vi "AD5933_ReadFrequencySweepValues (NI-845x I2C)(SubVI).vi"(7 "error in":errorcluster, 9 "ConfigRegister (0x80)":u8, 10 "NI-845x Config for I2C (in)":cluster{"i2c configuration":T1, "Refnum in":T2}) -> (0 "error out":errorcluster, 1 "I Array":i16[](array[numeric]), 2 "R Array":i16[](array[numeric]), 3 "NI-845x Config for I2C (out)":T3)   [LabVIEW 2017]
uses:
  <vilib>/ni845x/ni845x.llb/ni845xI2cConfiguration.ctl
  <vilib>/ni845x/ni845x.llb/ni845xControl.ctl
  TypeDefs/AD5933_CommandCodes.ctl
  TypeDefs/AD5933_Registers.ctl
  TypeDefs/AD5933_OperationState.ctl
  <vilib>/MakerHub/Toolbox/LMH-Toolbox.lvlib
panel:
  out "Frequency sweep complete":bool
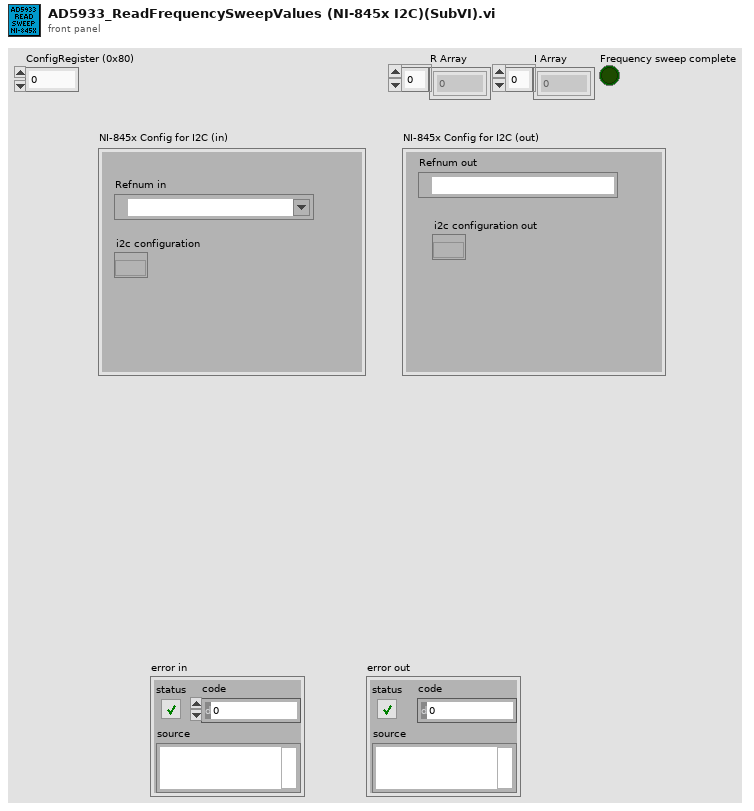
[diagram p1: front panel]
types:
  T1 = typedef "ni845xI2cConfiguration.ctl" = refnum<k20>
  T2 = typedef "ni845xControl.ctl" = refnum<k21>
  T3 = cluster{"i2c configuration out":T1, "Refnum out":T2}
  T4 = cluster{"Valid temperature measurement":bool, "Valid real/imaginary data":bool, "Frequency sweep complete":bool}
  T5 = typedef "AD5933_CommandCodes.ctl" = u8
  T6 = typedef "AD5933_Registers.ctl" = u8
  T7 = typedef "AD5933_OperationState.ctl" = u8
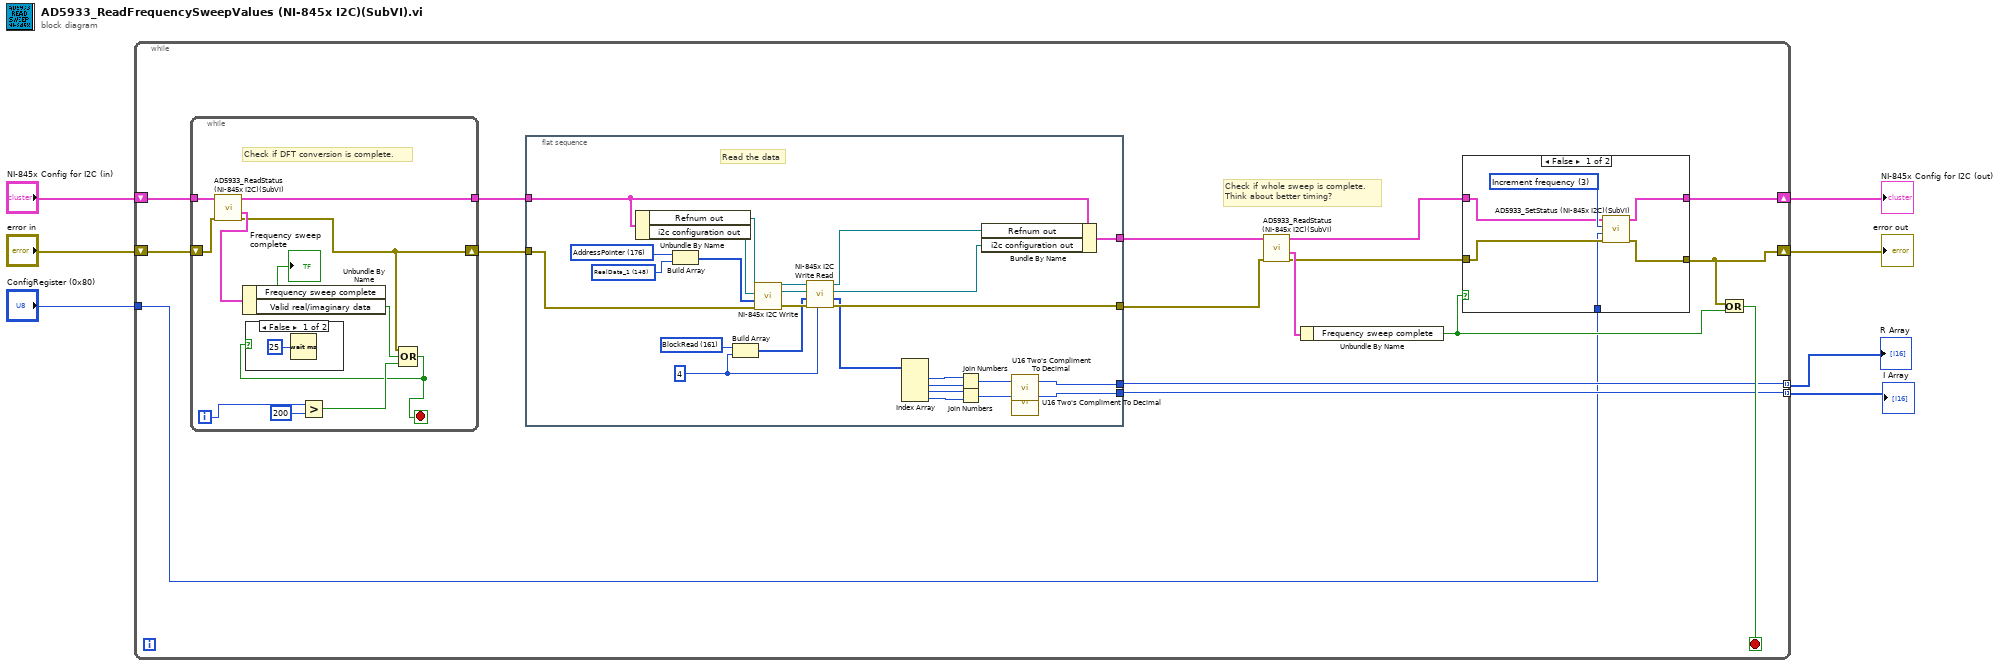
[diagram p0: block diagram]
diagram:
  n1 = while {
    shift-right: [w9] -> w6
    shift-left: "NI-845x Config for I2C (in)" -> [w16]
    shift-right: [w12] -> w4
    shift-left: "error in" -> [w21]
    tunnel: [w15] -> w3 mode=indexing
    tunnel: [w14] -> w2 mode=indexing
    tunnel: "ConfigRegister (0x80)" -> [w8]
    stop <- w17 stop-if-true
    # "Check if whole sweep is complete.\nThink about better timing?"
    n2 = while {
      tunnel: w16 -> [w68]
      tunnel: [w66] -> w23
      shift-right: [w61] -> w22
      shift-left: w21 -> [w63]
      i -> [w65]
      stop <- w58 stop-if-true
      # "Check if DFT conversion is complete."
      n3 = call "AD5933_ReadStatus (NI-845x I2C)(SubVI).vi"("error in"=w63, "NI-845x Config for I2C (in)"=w68) -> ("error out"=w61:errorcluster, "Status Info"=w67:T4, "NI-845x Config for I2C (out)"=w66:T3)  [unwired: 6 in]
      n4 = Unbundle By Name(w67) -> ("Frequency sweep complete"=→"Frequency sweep complete":bool, "Valid real/imaginary data"=w62:bool)
      n5 = Greater?(x=w65, y=200) -> (0:w60:bool)
      n6 = Compound Arithmetic op=OR(w61, w62, w60) -> (w58:bool)
      n7 = case shown="False" w58 {
        frame False {
          n8 = Wait (ms)(milliseconds to wait=u32 25) -> ()  [unwired: 1 out]
        }
        frame True {
        }
      }
    }
    n9 = flat-sequence {
      tunnel: [w51] -> w20
      tunnel: w23 -> [w48]
      tunnel: [w43] -> w19
      tunnel: w22 -> [w42]
      tunnel: [w33] -> w15
      tunnel: [w32] -> w14
      frame #0 {
        w37 = 4
        w47 = T5 161 items=["BlockWrite"=160, "BlockRead"=161, "AddressPointer"=176] ("CommandCodes")
        w49 = T6 148 items=["Control_1"=128, "Control_0"=129, "StartFeq_2"=130, "StartFeq_1"=131, "StartFeq_0"=132, "FreqInc_2"=133, "FreqInc_1"=134, "FreqInc_0"=135, "NumOfInc_1"=136, "NumOfInc_0"=137, "NumOfSetCycl_1"=138, "NumOfSetCycl_0"=139, "Status"=143, "TempData_1"=146, "TempData_0"=147, "RealData_1"=148, "RealData_0"=149, "ImagData_1"=150, "ImagData_0"=151] ("Register")
        w50 = T5 176 items=["BlockWrite"=160, "BlockRead"=161, "AddressPointer"=176] ("CommandCodes")
        # "Read the data"
        n10 = Unbundle By Name(w48) -> ("Refnum out"=w52:T2, "i2c configuration out"=w53:T1)
        n11 = Build Array(w50, w49) -> (w57:T6[])
        n12 = Build Array(w47, w37) -> (w46:i32[])
        n13 = call <vilib>:"NI-845x I2C Write.vi"("error in (no error)"=w42, "write data"=w57, "i2c configuration in"=w53, "device reference in"=w52) -> ("error out"=w56:errorcluster, "i2c configuration out"=w55:T1, "device reference out"=w54:T2)  [unwired: 5 in]
        n14 = call <vilib>:"NI-845x I2C Write Read.vi"("num bytes to read"=w37, "error in (no error)"=w56, "write data"=w46, "i2c configuration in"=w55, "device reference in"=w54) -> ("error out"=w43:errorcluster, "read data"=w36:u8[], "i2c configuration out"=w44:T1, "device reference out"=w45:T2)  [unwired: 3 in]
        n15 = Index Array(array=w36) -> (element #1=w41:u8, element #2=w40:u8, element #3=w39:u8, element #4=w38:u8)  [unwired: 4 in]
        n16 = Join Numbers(hi=w41, lo=w40) -> ((hi.lo)=w35:u16)
        n17 = Join Numbers(hi=w39, lo=w38) -> ((hi.lo)=w34:u16)
        n18 = Bundle By Name(cluster=w48, "Refnum out"=w45, "i2c configuration out"=w44) -> (w51:T3)
        n19 = call <vilib>:"U16 Two's Compliment To Decimal.vi"("Two's Compliment U16"=w35) -> ("Decimal I16"=w33:i16)  [unwired: 2 in]
        n20 = call <vilib>:"U16 Two's Compliment To Decimal.vi"("Two's Compliment U16"=w34) -> ("Decimal I16"=w32:i16)  [unwired: 2 in]
      }
    }
    n21 = call "AD5933_ReadStatus (NI-845x I2C)(SubVI).vi"("error in"=w19, "NI-845x Config for I2C (in)"=w20) -> ("error out"=w11:errorcluster, "Status Info"=w18:T4, "NI-845x Config for I2C (out)"=w10:T3)  [unwired: 6 in]
    n22 = Unbundle By Name(w18) -> ("Frequency sweep complete"=w13:bool)
    n23 = case shown="False" w13 {
      tunnel: [w26 w31] -> w12
      tunnel: w11 -> [w25 w31]
      tunnel: w10 -> [w28 w30]
      tunnel: [w27 w30] -> w9
      tunnel: w8 -> [w24 _]
      frame False {
        w29 = T7 3 items=["Initialize with start frequency"=1, "Start frequency sweep"=2, "Increment frequency"=3, "Repeat frequency"=4, "Measure temperature"=9, "Power-down mode"=10, "Standby mode"=11] ("ControlRegisterStates(D15-D12)")
        n24 = call "AD5933_SetStatus (NI-845x I2C)(SubVI).vi"("error in"=w25, "ConfigRegister (0x80)"=w24, "ControlRegisterStates(D15-D12)"=w29, "NI-845x Config for I2C (in)"=w28) -> ("error out"=w26:errorcluster, "NI-845x Config for I2C (out)"=w27:T3)  [unwired: 5 in]
      }
      frame True {
      }
    }
    n25 = Or(x=w12, y=w13) -> (x .or. y?=w17:bool)
  }
  "error out" <- w4
  "NI-845x Config for I2C (out)" <- w6
  "R Array" <- w3
  "I Array" <- w2
